vi "Guia-1 - Copia.vi"() -> ()   [LabVIEW 2014]
doc: "Newport Motion Controler\nThis VI test a Group\n\nAndré Romero - 2022\nandretec@ifsc.usp.br"
uses:
  <vilib>/Platform/TimedLoop/XDataNode/timing_clust.ctl
  <vilib>/Platform/TimedLoop/XDataNode/nitl_modes.ctl
  <vilib>/Platform/TimedLoop/XDataNode/wakeup.ctl
  <vilib>/Platform/TimedLoop/XDataNode/XDataNode.xnode
  <userlib>/Newport ESP301/Newport ESP301.lvlib
  <vilib>/Platform/TimedLoop/XDataNode/XDNodeRunTimeDep.lvlib
panel:
  in  "arc sweep angle 4":dbl=90.0 format="%#_13g"
  in  "arco volta 2 y_centro":dbl=-0.5 format="%#_13g"
  in  "arco volta 2 x_centro":dbl=5.0 format="%#_13g"
  in  "arco volta  1 x_centro":dbl=6.0 format="%#_13g"
  in  "arc sweep angle 3":dbl=-90.0 format="%#_13g"
  in  "arco volta 2 y_centro":dbl=-0.5 format="%#_13g"
  in  "Decceleration (mm/s²)":dbl=100.0 min=0.0 format="%.6g"
  in  "Acceleration (mm/s²)":dbl=100.0 min=0.0 format="%.6g"
  in  "arc sweep angle 2":dbl=90.0 format="%#_13g"
  in  "coordenada y_centro":dbl=-0.5 format="%#_13g"
  in  "coordenada x_centro":dbl=6.0 format="%#_13g"
  in  "coordenada x_centro":dbl=5.0 format="%#_13g"
  in  "arc sweep angle":dbl=-90.0 format="%#_13g"
  in  "coordenada y_centro":dbl=-0.5 format="%#_13g"
  in  "Stop Button":bool
  out "error out":errorcluster
  out "Y":dbl format="%.2g"
  out "X":dbl format="%.2f"
  out "XY Graph":cluster{dbl[], dbl[]}[](graph)
  in  "Velocity (mm/s)":dbl=0.1
  # "1o arco"
  # "2o arco"
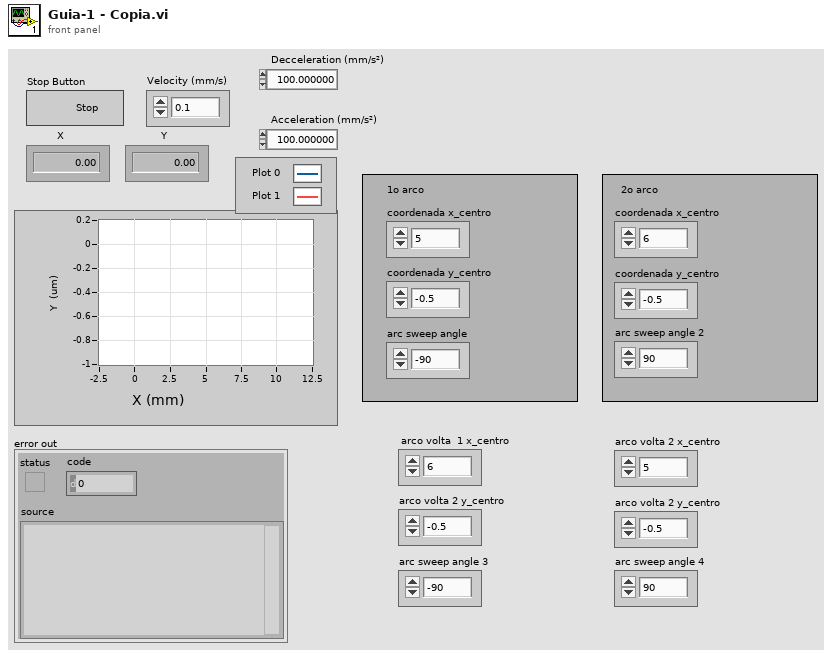
[diagram p1: front panel]
types:
  T1 = typedef "XDNodeRunTimeDep.lvlib/timing_clust.ctl" = cluster{"Expected End [f-1]":u64, "Actual End [f-1]":u64, "Finished Late? [f-1]":bool, "Expected End [i-1]":u64, "Actual End [i-1]":u64, "Finished Late? [i-1]":bool, "Expected Start [i]":u64, "Actual Start [i]":u64, "Expected Start [f]":u64, "Actual Start [f]":u64, "Source Name":string, "Structure Name":string, "Period":i64, "Deadline":i64, "Offset":i64, "Start":i64, "Priority":i32, "Timeout":i32, "Mode":T2, "Wakeup Reason":T3, "Error":errorcluster, "Source Type":string, "Secondary Source Type":string, "Global End Time":u64, "Global Start Time":u64, "Frame Duration":u64, "Iteration Duration":u64, "Assigned CPU":i32, "I/O Scan Engine Mode":u32}
  T2 = typedef "XDNodeRunTimeDep.lvlib/nitl_modes.ctl" = enum32{"No Change", "Process missed periods, maintain original phase", "Discard missed periods, maintain original phase", "Process missed periods, ignore original phase", "Discard missed periods, ignore original phase"}
  T3 = typedef "XDNodeRunTimeDep.lvlib/wakeup.ctl" = enum32{"Normal", "Aborted", "Asynchronous wakeup", "Timing source error", "Timed loop error", "Timeout"}
  T4 = cluster{"coordenada x_centro":dbl, "coordenada y_centro":dbl, "arc sweep angle":dbl}
  T5 = cluster{"coordenada x_centro":dbl, "coordenada y_centro":dbl, "arc sweep angle 2":dbl}
  T6 = cluster{"arco volta  1 x_centro":dbl, "arco volta 2 y_centro ":dbl, "arc sweep angle 3":dbl}
  T7 = cluster{"arco volta 2 x_centro":dbl, "arco volta 2 y_centro ":dbl, "arc sweep angle 4":dbl}
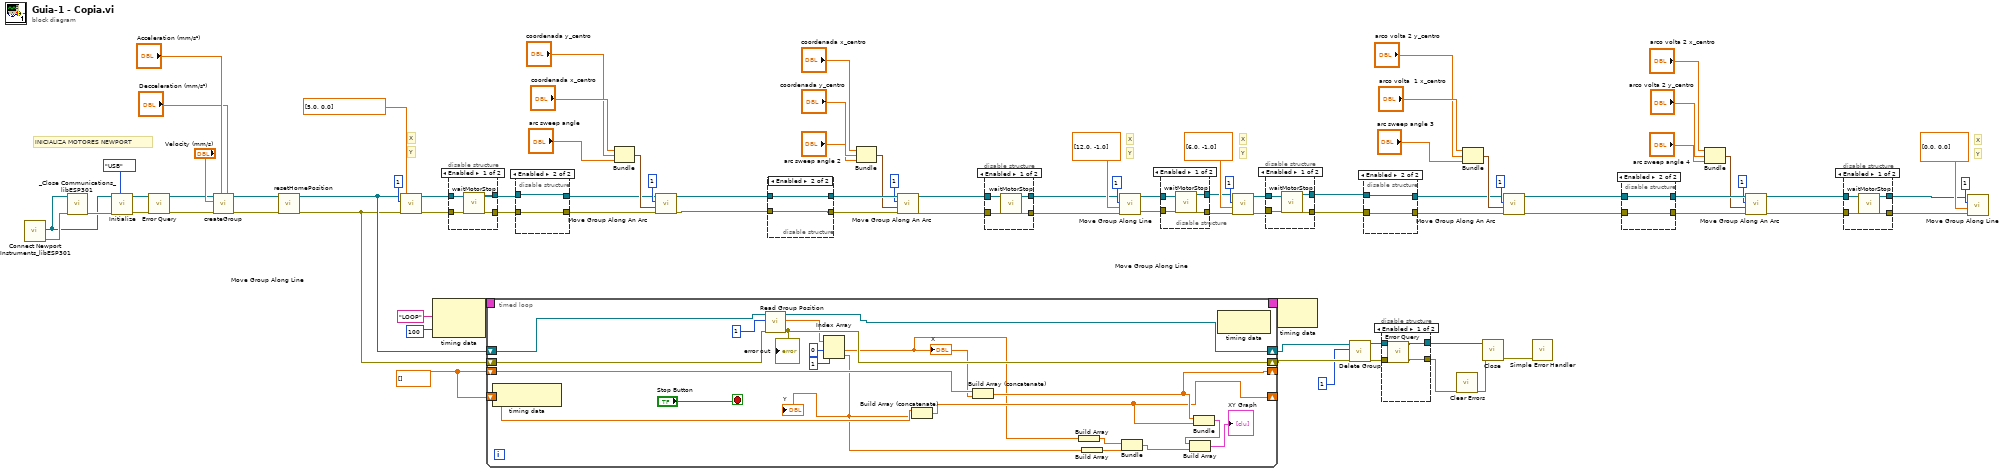
[diagram p0: block diagram]
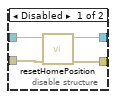
[diagram p5: hidden frame]
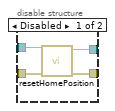
[diagram p8: hidden frame]
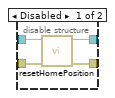
[diagram p9: hidden frame]
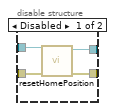
[diagram p10: hidden frame]
diagram:
  w72 = dbl[] []
  # "Y"
  # "X"
  # "Y"
  # "X"
  # "Y"
  # "X"
  # "Y"
  # "X"
  # "INICIALIZA MOTORES NEWPORT"
  n1 = call <userlib>:"Connect Newport Instruments_libESP301.vi"() -> ("error (duplicate)"=w85:errorcluster, "VISA resource name (duplicate)"=w84:refnum<visa-resource-name>)  [unwired: 7 in, 3 out]
  n2 = call <userlib>:"_Close Communications_libESP301.vi"("Instrument Channel"=w84, "error in (no error)"=w85) -> ("error out"=w87:errorcluster)  [unwired: 13 in]
  n3 = call <userlib>:"Initialize.vi"("VISA resource name"=w84, "error in (no error)"=w87, "Serial Link (RS232)"=enum16{"RS232", "USB"}."USB") -> ("VISA resource name out"=w83:refnum<visa-resource-name>, "error out"=w82:errorcluster)  [unwired: 6 in]
  n4 = call <userlib>:"Error Query.vi"("error in (no error)"=w82, "VISA resource name"=w83) -> ("error out"=w60:errorcluster, "VISA resource name out"=w61:refnum<visa-resource-name>)  [unwired: 2 in, 2 out]
  n5 = call "createGroup.vi"("Decceleration (0 units/s²)"="Decceleration (mm/s²)", "Acceleration (0 units/s²)"="Acceleration (mm/s²)", "error in (no error)"=w60, "Velocity"="Velocity (mm/s)", "VISA Refnum in"=w61) -> ("error out"=w47:errorcluster, "VISA Refnum out"=w46:refnum<visa-resource-name>)  [unwired: 5 in]
  n6 = call "resetHomePosition.vi"("error in (no error)"=w47, "VISA Refnum in"=w46) -> ("error out"=w44:errorcluster, "VISA Refnum out"=w45:refnum<visa-resource-name>)  [unwired: 8 in]
  n7 = call <userlib>:"Move Group Along Line.vi"("error in (no error)"=w44, "Position (0 units)"=dbl[] [5.0, 0.0], "Group Number (1)"=1, "VISA resource name"=w45) -> ("error out"=w14:errorcluster, "VISA resource name out"=w15:refnum<visa-resource-name>)  [unwired: 2 in]
  n8 = node-c288("LOOP" ("Structure Name"), i64 100 ("Period")) -> (w76:T1)
  n9 = disable-structure shown="Enabled" {
    disable-tunnel: [w91 w93] -> _
    disable-tunnel: [w90 w92] -> _
    disable-tunnel: w15 -> [w89 _]
    disable-tunnel: w14 -> [w88 _]
    frame Enabled {
      n10 = call "waitMotorStop.vi"("error in (no error)"=w88, "VISA Refnum in"=w89) -> ("error out"=w90:errorcluster, "VISA Refnum out"=w91:refnum<visa-resource-name>)  [unwired: 8 in]
    }
    frame Disabled {
    }
  }
  n11 = timed-loop {
    timing: w76 -> [_]
    timing-out: [_] -> w75
    shift-right: [w108] -> w67
    shift-left: w45 -> [w110]
    shift-right: [w107] -> w66
    shift-left: w44 -> [w109]
    shift-right: [w102] -> _
    shift-left: w72 -> [w113]
    shift-right: [w101] -> _
    shift-left: w72 -> [w112]
    stop <- "Stop Button" stop-if-true
    n12 = node-c288() -> ()  [unwired: 1 in, 1 out]
    n13 = call <userlib>:"Read Group Position.vi"("error in (no error)"=w109, "Group Number (1)"=1, "VISA resource name"=w110) -> ("error out"=w107:errorcluster, "Position (units)"=w104:dbl[], "VISA resource name out"=w108:refnum<visa-resource-name>)  [unwired: 2 in]
    "error out" <- w107
    n14 = Index Array(array=w104, index #1=0 ("index"), index #2=1 ("index")) -> (element #1=w95:dbl, element #2=w94:dbl)
    "Y" <- w94
    "X" <- w95
    n15 = Build Array (concatenate)(w112, w94) -> (w101:dbl[])
    n16 = Build Array (concatenate)(w113, w95) -> (w102:dbl[])
    n17 = Build Array(w95) -> (w97:dbl[])
    n18 = Build Array(w94) -> (w96:dbl[])
    n19 = Bundle(w97, w96) -> (w98:cluster{dbl[], dbl[]})  [unwired: 1 in]
    n20 = Bundle(w102, w101) -> (w100:cluster{dbl[], dbl[]})  [unwired: 1 in]
    n21 = Build Array(w100, w98) -> (→"XY Graph":cluster{dbl[], dbl[]}[])
    n22 = node-c288() -> ()  [unwired: 1 in, 1 out]
  }
  n23 = disable-structure shown="Enabled" {
    disable-tunnel: [w119 w121] -> w59
    disable-tunnel: [w118 w120] -> w58
    disable-tunnel: w15 -> [w117 w121]
    disable-tunnel: w14 -> [w116 w120]
    frame Disabled {
      n24 = call "resetHomePosition.vi"("error in (no error)"=w116, "VISA Refnum in"=w117) -> ("error out"=w118:errorcluster, "VISA Refnum out"=w119:refnum<visa-resource-name>)  [unwired: 8 in]
    }
    frame Enabled {
    }
  }
  n25 = Bundle("coordenada x_centro"="coordenada x_centro", "coordenada y_centro"="coordenada y_centro", "arc sweep angle"="arc sweep angle") -> (w77:T4)  [unwired: 1 in]
  n26 = call <userlib>:"Move Group Along An Arc.vi"("error in (no error)"=w58, "Arc  Parameters"=w77, "Group Number (1)"=1, "VISA resource name"=w59) -> ("error out"=w20:errorcluster, "VISA resource name out"=w21:refnum<visa-resource-name>)  [unwired: 2 in]
  n27 = disable-structure shown="Enabled" {
    disable-tunnel: [w125 w127] -> w57
    disable-tunnel: [w124 w126] -> w56
    disable-tunnel: w21 -> [w123 w127]
    disable-tunnel: w20 -> [w122 w126]
    frame Disabled {
      n28 = call "resetHomePosition.vi"("error in (no error)"=w122, "VISA Refnum in"=w123) -> ("error out"=w124:errorcluster, "VISA Refnum out"=w125:refnum<visa-resource-name>)  [unwired: 8 in]
    }
    frame Enabled {
    }
  }
  n29 = Bundle("coordenada x_centro"="coordenada x_centro", "coordenada y_centro"="coordenada y_centro", "arc sweep angle 2"="arc sweep angle 2") -> (w50:T5)  [unwired: 1 in]
  n30 = call <userlib>:"Move Group Along An Arc.vi"("error in (no error)"=w56, "Arc  Parameters"=w50, "Group Number (1)"=1, "VISA resource name"=w57) -> ("error out"=w7:errorcluster, "VISA resource name out"=w8:refnum<visa-resource-name>)  [unwired: 2 in]
  n31 = disable-structure shown="Enabled" {
    disable-tunnel: [w131 w133] -> w6
    disable-tunnel: [w130 w132] -> w5
    disable-tunnel: w8 -> [w129 w133]
    disable-tunnel: w7 -> [w128 w132]
    frame Enabled {
      n32 = call "waitMotorStop.vi"("error in (no error)"=w128, "VISA Refnum in"=w129) -> ("error out"=w130:errorcluster, "VISA Refnum out"=w131:refnum<visa-resource-name>)  [unwired: 8 in]
    }
    frame Disabled {
    }
  }
  n33 = call <userlib>:"Move Group Along Line.vi"("error in (no error)"=w5, "Position (0 units)"=dbl[] [12.0, -1.0], "Group Number (1)"=1, "VISA resource name"=w6) -> ("error out"=w11:errorcluster, "VISA resource name out"=w12:refnum<visa-resource-name>)  [unwired: 2 in]
  n34 = disable-structure shown="Enabled" {
    disable-tunnel: [w137 w138] -> w9
    disable-tunnel: w12 -> [w136 w139]
    disable-tunnel: w11 -> [w135 w138]
    disable-tunnel: [w134 w139] -> w10
    frame Enabled {
      n35 = call "waitMotorStop.vi"("error in (no error)"=w135, "VISA Refnum in"=w136) -> ("error out"=w137:errorcluster, "VISA Refnum out"=w134:refnum<visa-resource-name>)  [unwired: 8 in]
    }
    frame Disabled {
    }
  }
  n36 = call <userlib>:"Move Group Along Line.vi"("error in (no error)"=w9, "Position (0 units)"=dbl[] [6.0, -1.0], "Group Number (1)"=1, "VISA resource name"=w10) -> ("error out"=w18:errorcluster, "VISA resource name out"=w19:refnum<visa-resource-name>)  [unwired: 2 in]
  n37 = disable-structure shown="Enabled" {
    disable-tunnel: w19 -> [w143 w145]
    disable-tunnel: w18 -> [w142 w144]
    disable-tunnel: [w141 w145] -> w16
    disable-tunnel: [w140 w144] -> w17
    frame Enabled {
      n38 = call "waitMotorStop.vi"("error in (no error)"=w142, "VISA Refnum in"=w143) -> ("error out"=w140:errorcluster, "VISA Refnum out"=w141:refnum<visa-resource-name>)  [unwired: 8 in]
    }
    frame Disabled {
    }
  }
  n39 = node-c288(w75) -> ()  [unwired: 1 out]
  n40 = call <userlib>:"Delete Group.vi"("error in (no error)"=w66, "Group Number (1)"=1, "VISA resource name"=w67) -> ("error out"=w70:errorcluster, "VISA resource name out"=w71:refnum<visa-resource-name>)  [unwired: 3 in]
  n41 = disable-structure shown="Enabled" {
    disable-tunnel: [w149 w151] -> w36
    disable-tunnel: [w148 w150] -> w35
    disable-tunnel: w16 -> [w147 w151]
    disable-tunnel: w17 -> [w146 w150]
    frame Disabled {
      n42 = call "resetHomePosition.vi"("error in (no error)"=w146, "VISA Refnum in"=w147) -> ("error out"=w148:errorcluster, "VISA Refnum out"=w149:refnum<visa-resource-name>)  [unwired: 8 in]
    }
    frame Enabled {
    }
  }
  n43 = disable-structure shown="Enabled" {
    disable-tunnel: w71 -> [w155 w157]
    disable-tunnel: w70 -> [w154 w156]
    disable-tunnel: [w153 w157] -> w69
    disable-tunnel: [w152 w156] -> w64
    frame Enabled {
      n44 = call <userlib>:"Error Query.vi"("error in (no error)"=w154, "VISA resource name"=w155) -> ("error out"=w152:errorcluster, "VISA resource name out"=w153:refnum<visa-resource-name>)  [unwired: 2 in, 2 out]
    }
    frame Disabled {
    }
  }
  n45 = call <vilib>:"Clear Errors.vi"("error in (no error)"=w64) -> ("error out"=w63:errorcluster)  [unwired: 5 in, 1 out]
  n46 = Bundle("arco volta  1 x_centro"="arco volta  1 x_centro", "arco volta 2 y_centro"="arco volta 2 y_centro", "arc sweep angle 3"="arc sweep angle 3") -> (w37:T6)  [unwired: 1 in]
  n47 = call <userlib>:"Close.vi"("error in (no error)"=w63, "VISA resource name"=w69) -> ("error out"=w68:errorcluster)  [unwired: 9 in]
  n48 = call <userlib>:"Move Group Along An Arc.vi"("error in (no error)"=w35, "Arc  Parameters"=w37, "Group Number (1)"=1, "VISA resource name"=w36) -> ("error out"=w22:errorcluster, "VISA resource name out"=w23:refnum<visa-resource-name>)  [unwired: 2 in]
  n49 = call <vilib>:"Simple Error Handler.vi"("error in (no error)"=w68) -> ()  [unwired: 4 in, 5 out]
  n50 = disable-structure shown="Enabled" {
    disable-tunnel: [w161 w163] -> w34
    disable-tunnel: [w160 w162] -> w33
    disable-tunnel: w22 -> [w159 w162]
    disable-tunnel: w23 -> [w158 w163]
    frame Disabled {
      n51 = call "resetHomePosition.vi"("error in (no error)"=w159, "VISA Refnum in"=w158) -> ("error out"=w160:errorcluster, "VISA Refnum out"=w161:refnum<visa-resource-name>)  [unwired: 8 in]
    }
    frame Enabled {
    }
  }
  n52 = Bundle("arco volta 2 x_centro"="arco volta 2 x_centro", "arco volta 2 y_centro"="arco volta 2 y_centro", "arc sweep angle 4"="arc sweep angle 4") -> (w26:T7)  [unwired: 1 in]
  n53 = call <userlib>:"Move Group Along An Arc.vi"("error in (no error)"=w33, "Arc  Parameters"=w26, "Group Number (1)"=1, "VISA resource name"=w34) -> ("error out"=w3:errorcluster, "VISA resource name out"=w4:refnum<visa-resource-name>)  [unwired: 2 in]
  n54 = disable-structure shown="Enabled" {
    disable-tunnel: [w167 w169] -> w2
    disable-tunnel: [w166 w168] -> w1
    disable-tunnel: w4 -> [w165 w169]
    disable-tunnel: w3 -> [w164 w168]
    frame Enabled {
      n55 = call "waitMotorStop.vi"("error in (no error)"=w164, "VISA Refnum in"=w165) -> ("error out"=w166:errorcluster, "VISA Refnum out"=w167:refnum<visa-resource-name>)  [unwired: 8 in]
    }
    frame Disabled {
    }
  }
  n56 = call <userlib>:"Move Group Along Line.vi"("error in (no error)"=w1, "Position (0 units)"=dbl[] [0.0, 0.0], "Group Number (1)"=1, "VISA resource name"=w2) -> ()  [unwired: 2 in, 2 out]
